vi "set_number_of_rois.vi"(8 "error in (no error)":errorcluster, 10 "number of ROIs":i32, 11 "TrajectoryDL121017Hopping in":refnum<class "TrajectoryDL121017Hopping.lvclass">) -> (0 "error out":errorcluster, 3 "TrajectoryDL121017Hopping out":refnum<class "TrajectoryDL121017Hopping.lvclass">)   [LabVIEW 2010, in "TrajectoryDL121017Hopping.lvclass"]
uses:
  TrajectoryDL121017Hopping.lvclass
  TrajectoryDL121017Hopping.lvclass/TrajectoryDL121017Hopping.ctl
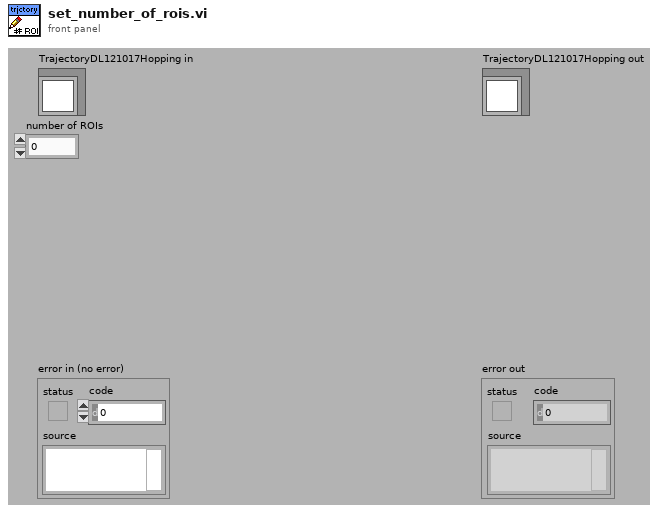
[diagram p1: front panel]
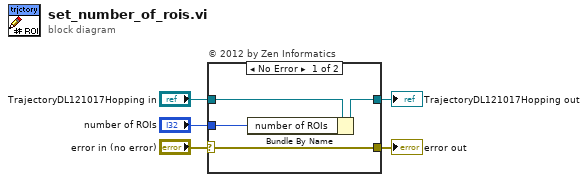
[diagram p0: block diagram]
diagram:
  n1 = case "© 2012 by Zen Informatics" shown="No Error" "error in (no error)" {
    selector: "error in (no error)" -> [w9 w11]
    tunnel: [w9 w11] -> w4
    tunnel: [w7 w10] -> w2
    tunnel: "TrajectoryDL121017Hopping in" -> [w8 w10]
    tunnel: "number of ROIs" -> [w6 _]
    frame No Error {
      n2 = Bundle By Name(cluster=w8, "number of ROIs"=w6) -> (w7:refnum<class "TrajectoryDL121017Hopping.lvclass">)
    }
    frame Error {
    }
  }
  "error out" <- w4
  "TrajectoryDL121017Hopping out" <- w2
